vi "Get Instrument Names.vi"(1 "Instrument List":T1[](array[typedef]) {"Status" format="%.0x"}) -> (0 "Names":T2[](array[typedef]))   [LabVIEW 2024]
uses:
  Sub Controls/Instrument Info.ctl
  Sub Controls/Instrument IDN.ctl
  Sub Controls/Instrument Actions.ctl
  Sub Controls/Instrument Ref.ctl
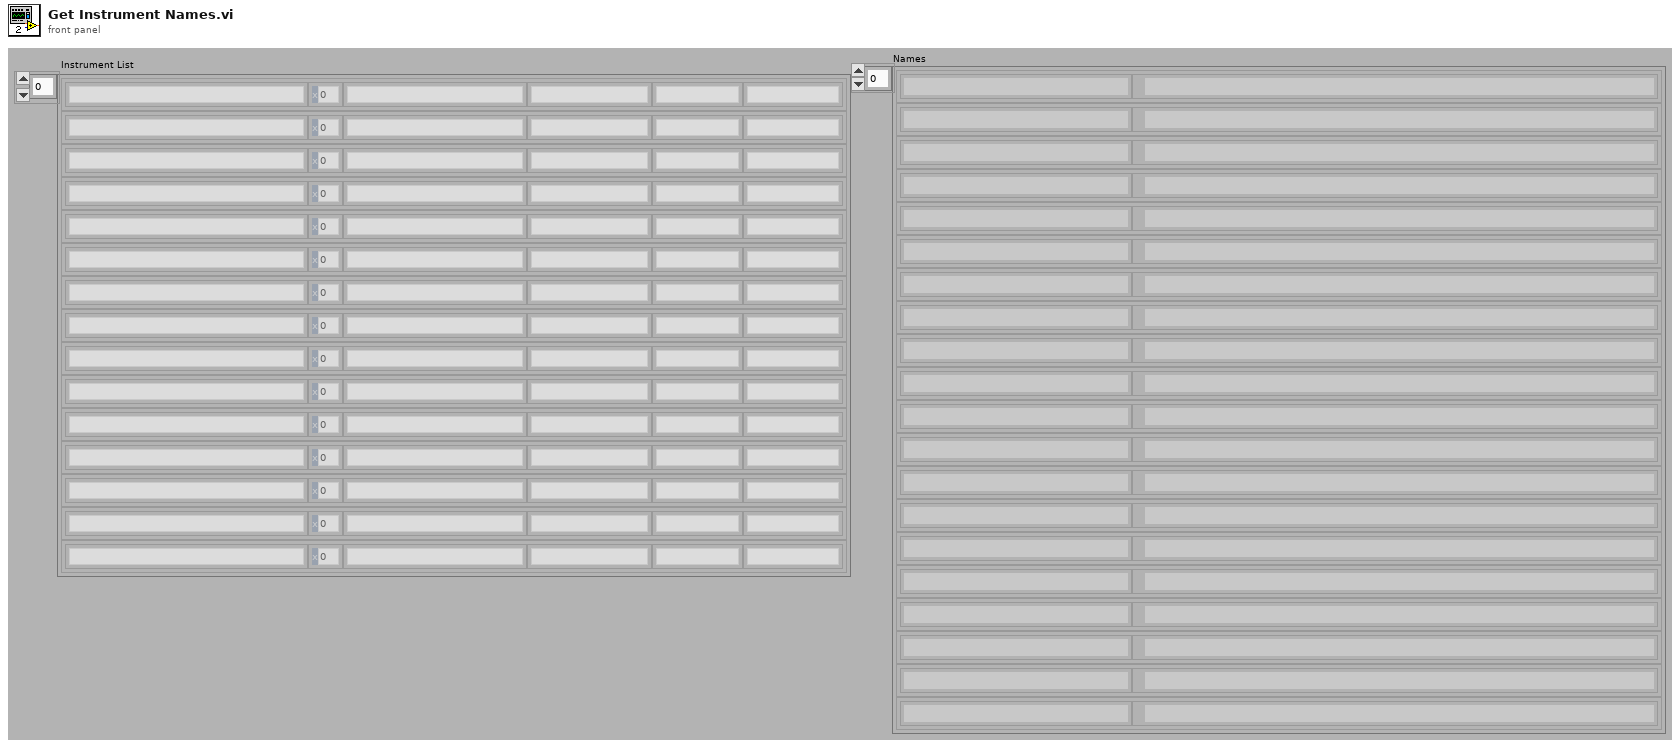
[diagram p1: front panel]
types:
  T1 = typedef "Instrument IDN.ctl" = cluster{"VISA Address":string, "Status":u16, "Manufacturer":string, "Model":string, "Info":string, "Info 2":string, "Misc Data":variant}
  T2 = typedef "Instrument Info.ctl" = cluster{"Name":string, "path":path}
  T3 = typedef "Instrument Actions.ctl" = enum16{"Scan", "Identify", "New", "Configure", "Initialize", "Test", "Read", "Close"}
  T4 = typedef "Instrument Ref.ctl" = refnum<vi>
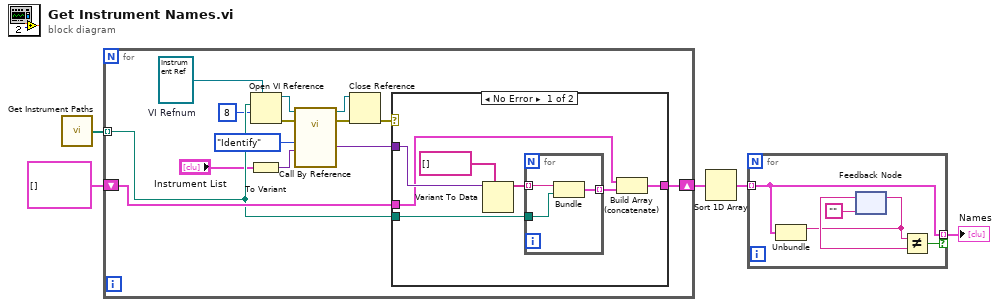
[diagram p0: block diagram]
diagram:
  n1 = call "Get Instrument Paths.vi"() -> ("paths"=w5:path[])  [unwired: 1 in]
  n2 = for {
    tunnel: w5 -> [w9] mode=indexing
    shift-right: [w16] -> w3
    shift-left: T2[] [] -> [w15]
    w10 = T4 refnum  # VI Refnum
    n3 = Open VI Reference(type specifier VI Refnum (for type only)=w10, vi path=w9, options=8) -> (vi reference=w19:T4, error out=w18:errorcluster)  [unwired: 3 in]
    n4 = To Variant(anything="Instrument List") -> (Variant=w7:variant)
    n5 = call-by-ref "?"(reference=w19, error in=w18, "Action"=Instrument_Actions."Identify", "Parameters"=w7) -> (reference out=w12:T4, error out=w14:errorcluster, "Output"=w17:variant)  [unwired: 4 in, 1 out]
    n6 = Close Reference(reference=w12, error in (no error)=w14) -> (error out=w13:errorcluster)
    n7 = case shown="No Error" w13 {
      tunnel: w17 -> [w26 _]
      tunnel: w9 -> [w25 _]
      tunnel: [w24 w30] -> w16
      tunnel: w15 -> [w22 w30]
      frame No Error {
        n8 = Variant To Data(type=string[] [], Variant=w26) -> (data=w21:string[])  [unwired: 1 in, 1 out]
        n9 = for {
          tunnel: w25 -> [w27]
          tunnel: [w29] -> w23 mode=indexing
          tunnel: w21 -> [w28] mode=indexing
          n10 = Bundle(w28, "appended path"=w27) -> (w29:cluster{string, "appended path":path})  [unwired: 1 in]
        }
        n11 = Build Array (concatenate)(w22, w23) -> (w24:T2[])
      }
      frame Error {
      }
    }
  }
  n12 = Sort 1D Array(array=w3) -> (sorted array=w2:T2[])
  n13 = for {
    tunnel: w2 -> [w35] mode=indexing
    tunnel: [w35] -> w1 mode=indexing if=w32
    n14 = Unbundle(w35) -> ("Name"=w33:string)  [unwired: 1 out]
    n15 = feedback-in #1(w33) -> ()
    n16 = feedback #1("") -> (w34:string)
    n17 = Not Equal?(x=w33, y=w34) -> (x != y?=w32:bool)
  }
  "Names" <- w1
